vi "getNextToCompile.vi"(8 "error in (no error)":errorcluster, 11 "Compiler in":refnum<class "Compiler.lvclass">) -> (0 "error out":errorcluster, 1 "newScript?":bool=TRUE, 2 "Path":path, 3 "Compiler out":refnum<class "Compiler.lvclass">)   [LabVIEW 2011, in "Compiler.lvlib" / "Compiler.lvclass"]
uses:
  Compiler.lvclass
  Compiler.lvclass/Compiler.ctl
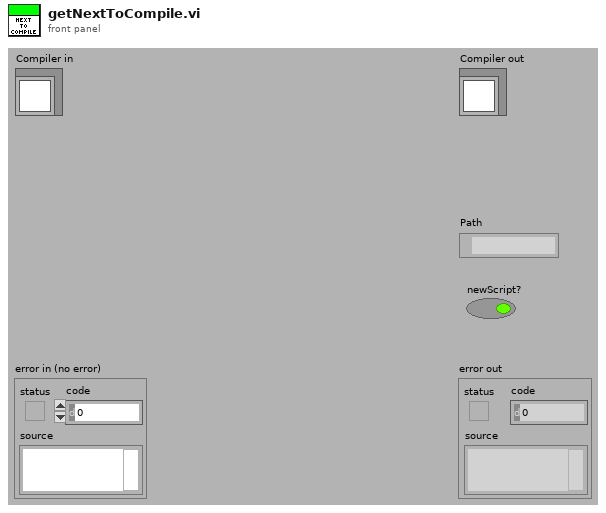
[diagram p1: front panel]
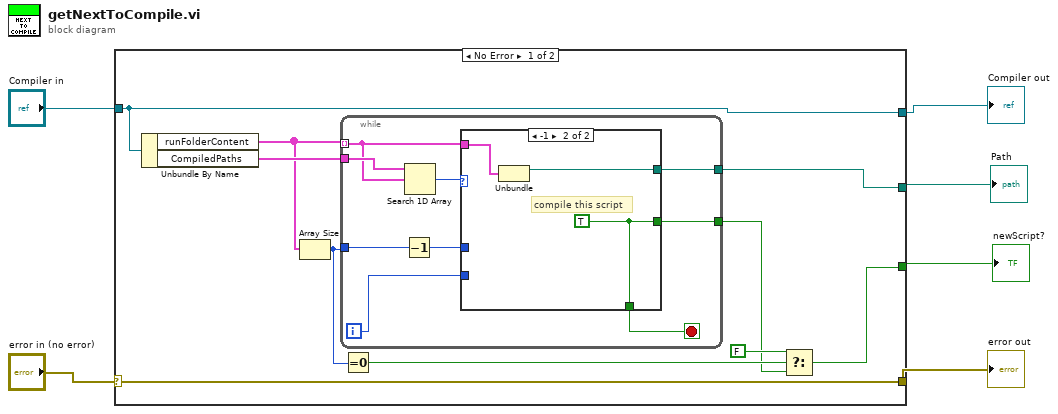
[diagram p0: block diagram]
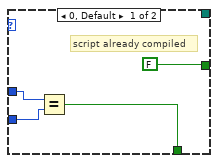
[diagram p2: hidden frame]
diagram:
  n1 = case shown="No Error" "error in (no error)" {
    selector: "error in (no error)" -> [w11 w34]
    tunnel: [w11 w34] -> w5
    tunnel: [w13 w33] -> w3
    tunnel: "Compiler in" -> [w13 w33]
    tunnel: [w7 _] -> w2
    tunnel: [w14 _] -> w1
    frame No Error {
      n2 = Unbundle By Name(w13) -> ("runFolderContent"=w15:cluster{path, "last mod":timestamp}[], "CompiledPaths"=w16:cluster{path, "lastCompiled":timestamp}[])
      n3 = Array Size(array=w15) -> (size(s)=w12:i32)
      n4 = while {
        tunnel: w15 -> [w23] mode=indexing
        tunnel: w16 -> [w25]
        tunnel: [w22] -> w14
        tunnel: w12 -> [w20]
        tunnel: [w18] -> w8
        i -> [w17]
        stop <- w21 stop-if-true
        n5 = Decrement(x=w20) -> (x-1=w19:i32)
        n6 = Search 1D Array(1D array=w25, element=w23) -> (index of element=w24:i32)  [unwired: 1 in]
        n7 = case shown="-1" w24 {
          tunnel: w23 -> [_ w32]
          tunnel: [_ w31] -> w22
          tunnel: [w27 w30] -> w21
          tunnel: w19 -> [w29 _]
          tunnel: w17 -> [w28 _]
          tunnel: [FALSE w30] -> w18
          frame 0, Default {
            # "script already compiled"
            n8 = Equal?(x=w29, y=w28) -> (x = y?=w27:bool)
          }
          frame -1 {
            w30 = TRUE
            # "compile this script"
            n9 = Unbundle(w32) -> (w31:path)  [unwired: 1 out]
          }
        }
      }
      n10 = Equal To 0?(x=w12) -> (x = 0?=w10:bool)
      n11 = Select(t=FALSE, s=w10, f=w8) -> (s? t:f=w7:bool)
    }
    frame Error {
    }
  }
  "error out" <- w5
  "Compiler out" <- w3
  "Path" <- w1
  "newScript?" <- w2
